vi "MCB2400 PWM PrjAttrValidator.vi"(5 "Attr Refnum":refnum<vi>, 9 "PWMNum (0-11)":u8(ring) items=["137", "138", "139", "140", "141", "142"], 11 "Attributes":T1={"Polarity"=FALSE, "Frequency (Hz)"=1000, "Programmable Pin Connections"=0} {"Programmable Pin Connections" items=["PWM0_1 uses pin P3.16. You can not use PWM0_1 and pin P2.0 in the same project.", "PWM0_2 uses pin P3.17. You can not use PWM0_2 and pin P2.1 in the same project.", "PWM0_3 uses pin P3.18. You can not use PWM0_3 and pin P2.2 in the same project.", "PWM0_4 uses pin P3.19. You can not use PWM0_4 and pin P2.3 in the same project.", "PWM0_5 uses pin P3.20. You can not use PWM0_5 and pin P2.4 in the same project.", "PWM0_6 uses pin P3.21. You can not use PWM0_6 and pin P2.5 in the same project.", "PWM1_1 uses pin P2.0. You can not use PWM1_1 and P3.16 in the same project.", "PWM1_2 uses pin P2.1. You can not use PWM1_2 and P3.17 in the same project.", "PWM1_3 uses pin P2.2. You can not use PWM1_3 and P3.18 in the same project.", "PWM1_4 uses pin P2.3. You can not use PWM1_4 and P3.19 in the same project.", "PWM1_5 uses pin P2.4. You can not use PWM1_5 and P3.20 in the same project.", "PWM1_6 uses pin P2.5. You can not use PWM1_6 and P3.21 in the same project."]}) -> (3 "Valid?":bool)   [LabVIEW 2011]
uses:
  <vilib>/Embedded/ARM/MCB2400/MCB2400_PWM_PrjAttr.ctl
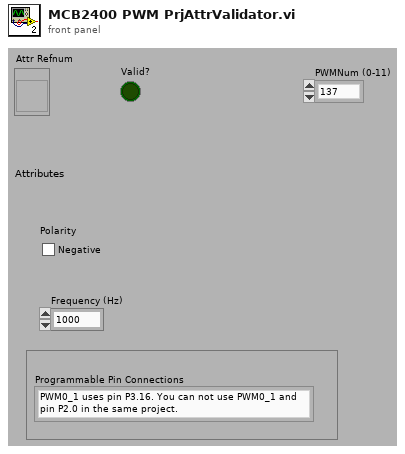
[diagram p1: front panel]
types:
  T1 = typedef "MCB2400_PWM_PrjAttr.ctl" = cluster{"Polarity":bool, "Frequency (Hz)":u32, "Programmable Pin Connections":u16}
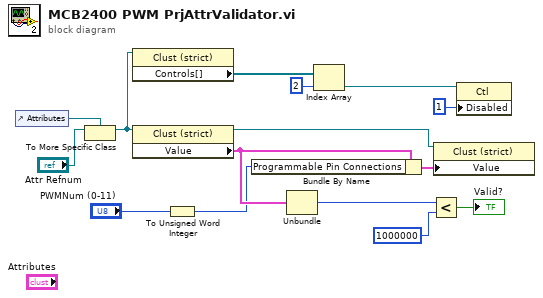
[diagram p0: block diagram]
diagram:
  n1 = control-ref of="Attributes"() -> (w2:refnum<vi>)
  n2 = To More Specific Class(target class=w2, reference="Attr Refnum") -> (specific class reference=w11:refnum<vi>)  [unwired: 1 in, 1 out]
  n3 = property class="Clust (strict)"(reference=w11) -> ("Controls[]"=w8:refnum<vi>[])  [unwired: 1 in, 2 out]
  n4 = property class="Clust (strict)"(reference=w11) -> (reference out=w6:refnum<vi>, "Value"=w5:T1)  [unwired: 1 in, 1 out]
  n5 = To Unsigned Word Integer(number="PWMNum (0-11)") -> (unsigned 16bit integer=w4:u16)
  n6 = Bundle By Name(cluster=w5, "Programmable Pin Connections"=w4) -> (w10:T1)
  n7 = Unbundle(w5) -> ("Frequency (Hz)"=w3:u32)  [unwired: 2 out]
  n8 = Index Array(array=w8, index=2) -> (element=w13:refnum<vi>)
  n9 = Less?(x=w3, y=u32 1000000 ("upper limit")) -> (x < y?=→"Valid?":bool)
  n10 = property class="Clust (strict)"(reference=w6, "Value"=w10) -> ()  [unwired: 1 in, 2 out]
  n11 = property class="Ctl"(reference=w13, "Disabled"=u8 1) -> ()  [unwired: 1 in, 2 out]
